vi "_WSACleanup.vi"(8 "Error In":errorcluster) -> (0 "Error Out":errorcluster)   [LabVIEW 2018]
uses:
  ws2_32.dll
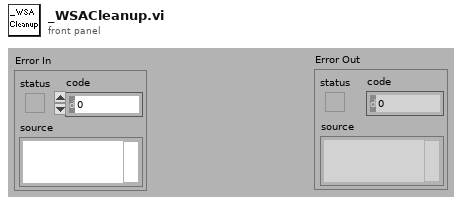
[diagram p1: front panel]
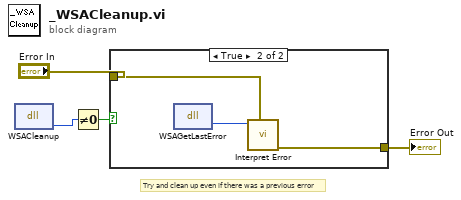
[diagram p0: block diagram]
diagram:
  # "Try and clean up even if there was a previous error"
  n1 = dll-call lib="ws2_32.dll" fn="WSACleanup"() -> (w4:i32)  [unwired: 3 in, 2 out]
  n2 = Not Equal To 0?(x=w4) -> (x != 0?=w3:bool)
  n3 = case shown="True" w3 {
    tunnel: "Error In" -> [w5 w7]
    tunnel: [w5 w6] -> w2
    frame False {
    }
    frame True {
      n4 = dll-call lib="ws2_32.dll" fn="WSAGetLastError"() -> (w8:i32)  [unwired: 3 in, 2 out]
      n5 = call "Interpret Error.vi"("Error In"=w7, "Code"=w8) -> ("Error Out"=w6:errorcluster)  [unwired: 9 in]
    }
  }
  "Error Out" <- w2
